vi "BuildMenu3.vi"(8 "Click Type":T1, 9 "Point":T2, 10 "XRef":refnum<vi>, 11 "State In":T10={"Input Type"=variant(dbl 0.0), "Selection"=0, "Element Names"=[], "Type Strings"=[], "Element Types"=[]}) -> (1 "Show Standard Items? (Popup click only)":bool=TRUE, 2 "Menu Specification":T4)   [LabVIEW 2015, in "Construct-Tagged-Union.xnode"]
doc: "This ability VI is used to describe the menu LabVIEW will display in response to a popup (right) click or a ShowMenu reply from OperateClick.\n \n Click Type is the type of click that led to this call of the ability. Point is the location of the user's popup click, and is relative to the top-left corner of your XNode's bounds. You may use this point to make your popup sensitive to the location that was clicked. Show Standard Items? is applicable only if Click Type is Popup, and tells LabVIEW whether it should include the standard popup items that are included on every node in LabVIEW.\n \n Menu Specification is an array of clusters describing the menu.\n Item: A string that will appear in the menu.\n Id: A string that identifies this item and will be passed to SelectMenu3.\n StartSub: The current string will be the header for a pull right menu.\n EndSub: The current string will be the last item in a pull right menu.\n Checked: The current item will have a check mark next to it.\n Disabled: The current item will be diabled and greyed out.\n Separator: The current item will be a separator. Item string is not displayed.\n Help: The text that should be displayed in context help when this menu item is hovered over. This functionality is currently not implemented.\n \n The index from this array will be an input to SelectMenu3.\n \n Remember to localize the strings in your menu.\n\nDefault behavior: Only show standard items for a popup click, show nothing for operate click.\n\nThis ability does not provide UI and OS messages are not handled.\n\nSee also: SelectMenu3"
uses:
  Construct-Tagged-Union.xnode
  State.ctl
  <vilib>/XNodeSupport/XNodeMenuSpecs3.ctl
  <vilib>/XNodeSupport/XNodeMenuSpec3.ctl
  <vilib>/XNodeSupport/XNodeString.ctl
  <vilib>/XNodeSupport/XNodeBool.ctl
  <vilib>/XNodeSupport/XNodeStandardHelpInfo.ctl
  <vilib>/XNodeSupport/XNodePath.ctl
  <vilib>/XNodeSupport/XNodePoint.ctl
  <vilib>/XNodeSupport/XNodeInt.ctl
  <vilib>/XNodeSupport/XNodeClickTypes.ctl
  <vilib>/XNodeSupport/NI_XNodeSupport.lvlib
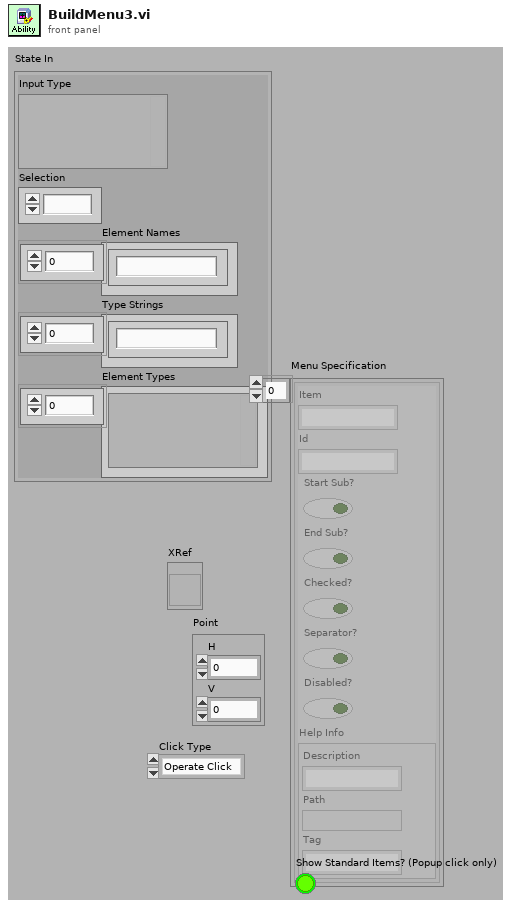
[diagram p1: front panel]
types:
  T1 = typedef "NI_XNodeSupport.lvlib/XNodeClickTypes.ctl" = enum32{"Operate Click", "Popup Click"}
  T2 = typedef "NI_XNodeSupport.lvlib/XNodePoint.ctl" = cluster{"H":T3, "V":T3}
  T3 = typedef "NI_XNodeSupport.lvlib/XNodeInt.ctl" = i32
  T4 = typedef "NI_XNodeSupport.lvlib/XNodeMenuSpecs3.ctl" = T5[]
  T5 = typedef "NI_XNodeSupport.lvlib/XNodeMenuSpec3.ctl" = cluster{"Item":T6, "Id":T6, "Start Sub?":T7, "End Sub?":T7, "Checked?":T7, "Separator?":T7, "Disabled?":T7, "Help Info":T8}
  T6 = typedef "NI_XNodeSupport.lvlib/XNodeString.ctl" = string
  T7 = typedef "NI_XNodeSupport.lvlib/XNodeBool.ctl" = bool
  T8 = typedef "NI_XNodeSupport.lvlib/XNodeStandardHelpInfo.ctl" = cluster{"Description":T6, "Path":T9, "Tag":T6}
  T9 = typedef "NI_XNodeSupport.lvlib/XNodePath.ctl" = path
  T10 = typedef "Construct-Tagged-Union.xnode/State.ctl" = cluster{"Input Type":variant, "Selection":i32, "Element Names":string[], "Type Strings":string[], "Element Types":variant[]}
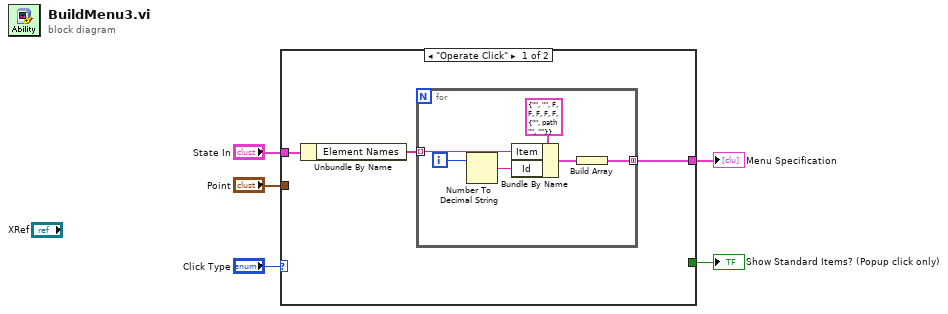
[diagram p0: block diagram]
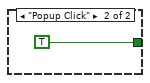
[diagram p2: hidden frame]
diagram:
  n1 = case shown="\"Operate Click\"" "Click Type" {
    tunnel: "State In" -> [w8 _]
    tunnel: [w6 _] -> w2
    tunnel: "Point" -> [_ _]
    tunnel: [_ TRUE] -> w1
    frame "Operate Click" {
      n2 = Unbundle By Name(w8) -> ("Element Names"=w7:string[])
      n3 = for {
        tunnel: w7 -> [w11] mode=indexing
        tunnel: [w12] -> w6 mode=concatenating
        i -> [w10]
        n4 = Number To Decimal String(number=w10) -> (decimal integer string=w9:string)  [unwired: 1 in]
        n5 = Bundle By Name(cluster=T5 {"Item"="", "Id"="", "Start Sub?"=FALSE, "End Sub?"=FALSE, "Checked?"=FALSE, "Separator?"=FALSE, "Disabled?"=FALSE, "Help Info"={"Description"="", "Path"=path "", "Tag"=""}} ("Menu Item 3"), "Item"=w11, "Id"=w9) -> (w13:T5)
        n6 = Build Array(w13) -> (w12:T5[])
      }
    }
    frame "Popup Click" {
    }
  }
  "Menu Specification" <- w2
  "Show Standard Items? (Popup click only)" <- w1
